vi "IMU RECORDER_AU_2024_v2.vi"() -> ()   [LabVIEW 2021]
uses:
  IMU data typedef.ctl
  <vilib>/Utility/sysdir.llb/System Directory Type.ctl
panel:
  out "TDMS REC!":bool
  in  "Run":bool caption="Run deluje le ob zagonu programa,\nda se zagotovi, da najprej izbereš port.\nÈe program ustaviš s tipko stop, moraš \nza ponoven zagon program še enkrat odpret."
  out "RT REC ID":i32
  in  "Tab Control 2":T1(tab)
  out "LostPackets":cluster{"f":dbl, "f":dbl}(graph)={"f"=1.0, "f"=1.0}
  out "LPR":cluster{dbl, dbl}(graph)={100.0, 100.0}
  out "BATT":cluster{"Ubat 1":dbl, "Ubat 2":dbl}(graph)
  out "Ubat 1":dbl
  out "IMU Temp 1":dbl=25.0
  out "DATA 1":string
  out "Stop IMU 1":bool
  in  "IMU port 1":u16=1235
  in  "T=last value, F=zero 1L":bool=TRUE
  out "Timeout 1":bool=TRUE
  out "IMU1 - 6D":refnum<k16>
  out "IMU DATA 1":T2
  out "IMU DATA 2":T2
  in  "IMU port 2":u16=2000
  out "DATA 2":string
  out "IMU2 - 6D":refnum<k16>
  in  "T=last value, F=zero 1L 2":bool=TRUE caption="T=last value, F=zero 1L"
  out "Timeout 2":bool=TRUE
  out "Stop IMU 2":bool
  out "LiPo MIN":dbl=3.4
  out "LiPo NOM":dbl=3.7
  out "F1":bool
  out "A1":bool=TRUE
  in  "stop 1":bool
  in  "stop 2":bool
  out "IMU Temp 2":dbl=25.0
  out "Ubat 2":dbl
  out "F2":bool
  out "A2":bool=TRUE
  out "GYRO 2":T3(graph)={"AVG(X,N)"=-1.87176, "AVG(X,N)"=2.10976, "AVG(X,N)"=1.55397}
  out "ACC 2":T3(graph)={"AVG(X,N)"=-0.0248636, "AVG(X,N)"=-0.031232, "AVG(X,N)"=0.0110239}
  out "GYRO 1":T3(graph)={"AVG(X,N)"=-1.87176, "AVG(X,N)"=1.48327, "AVG(X,N)"=2.96304}
  in  "IMU CHART":bool=TRUE
  in  "CAL IMU2":bool
  out "BIAS 1":T4={"ACCEL-X"=0.0236778, "ACCEL-Y"=0.0366586, "ACCEL-Z"=-0.00184464, "GYRO - X"=1.87176, "GYRO - Y"=-1.48327, "GYRO - Z"=-2.96304, "TIMESTAMP"=0.0}
  out "BIAS 2":T4={"ACCEL-X"=0.0248636, "ACCEL-Y"=0.031232, "ACCEL-Z"=-0.0110239, "GYRO - X"=1.87176, "GYRO - Y"=-2.10976, "GYRO - Z"=-1.55397, "TIMESTAMP"=0.0}
  out "ACC 1":T3(graph)={"AVG(X,N)"=-0.0236778, "AVG(X,N)"=-0.0366586, "AVG(X,N)"=0.00184464}
  in  "CAL IMU1":bool
  in  "N_BIAS_IMU":i32=100
  out "date/time string":string="2024_02_29"
  out "ShrambaLabview":path=path "C:/Users/marko/TDMS"
  out "Lokacija shranjevanja":path=path "C:/Users/marko/TDMS/2024_02_29"
  in  "sample time":u32=5
  out "LV TimeStamp":i32=16582790
  out "sample ID":i32=109936
  out "ovd":bool
  out "Seconds":i32=550 format="%.2f"
  out "REC FileName":string="IMU-06-06-18-13-48.tdms"
  out "TMP File Name":string="D-02-29-11-54-17.tdms"
  in  "RECORD":bool
  # "FSFV TAPING @ AU 2021 v2"
  # "IP address:  10.10.4.99"
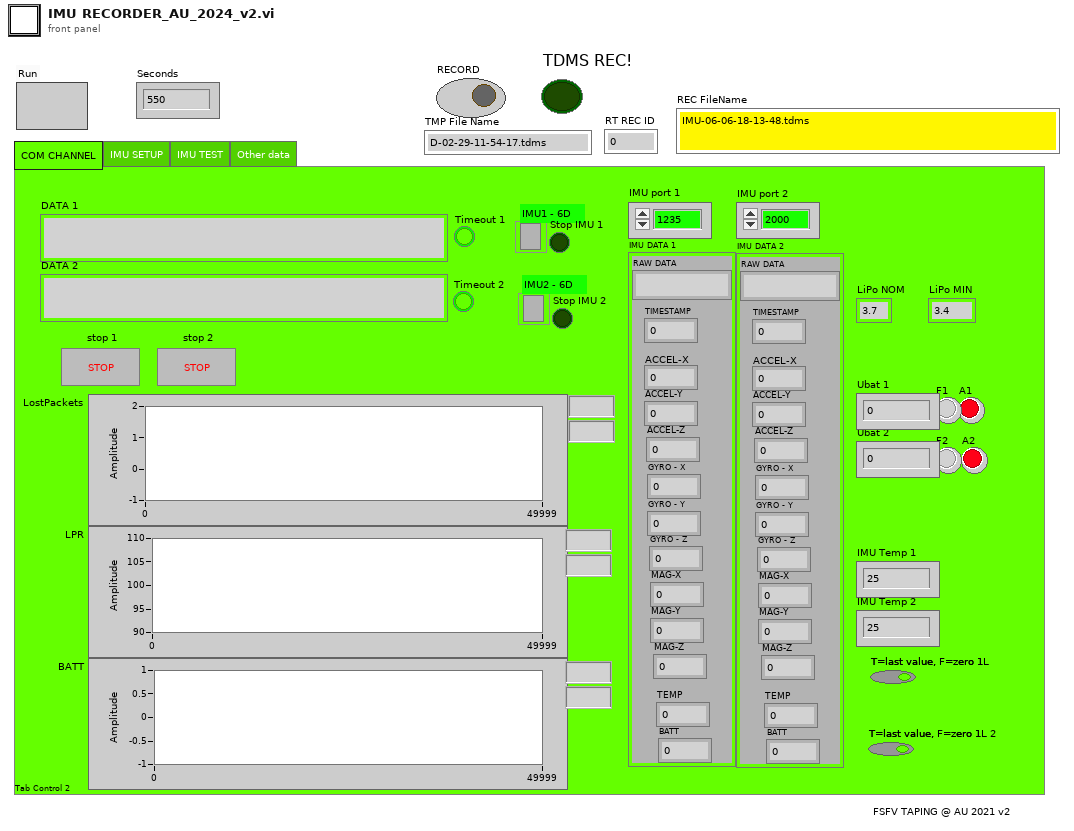
[diagram p1: front panel]
types:
  T1 = enum32{"COM CHANNEL", "IMU SETUP", "IMU TEST", "Other data"}
  T2 = typedef "IMU data typedef.ctl" = cluster{"ACCEL-X":dbl, "ACCEL-Y":dbl, "ACCEL-Z":dbl, "GYRO - X":dbl, "GYRO - Y":dbl, "GYRO - Z":dbl, "MAG-Z":dbl, "MAG-Y":dbl, "MAG-X":dbl, "TEMP":dbl, "BATT":dbl, "RAW DATA":string, "TIMESTAMP":dbl}
  T3 = cluster{"AVG(X,N)":dbl, "AVG(X,N)":dbl, "AVG(X,N)":dbl}
  T4 = cluster{"ACCEL-X":dbl, "ACCEL-Y":dbl, "ACCEL-Z":dbl, "GYRO - X":dbl, "GYRO - Y":dbl, "GYRO - Z":dbl, "TIMESTAMP":dbl}
  T5 = typedef "System Directory Type.ctl" = i32
  T6 = cluster{"ACCEL-X":dbl, "ACCEL-Y":dbl, "ACCEL-Z":dbl}
  T7 = cluster{"GYRO - X":dbl, "GYRO - Y":dbl, "GYRO - Z":dbl}
  T8 = cluster{"AVG(X,N)":dbl, "AVG(X,N)":dbl, dbl, "AVG(X,N)":dbl, "AVG(X,N)":dbl, "AVG(X,N)":dbl, "y":dbl}
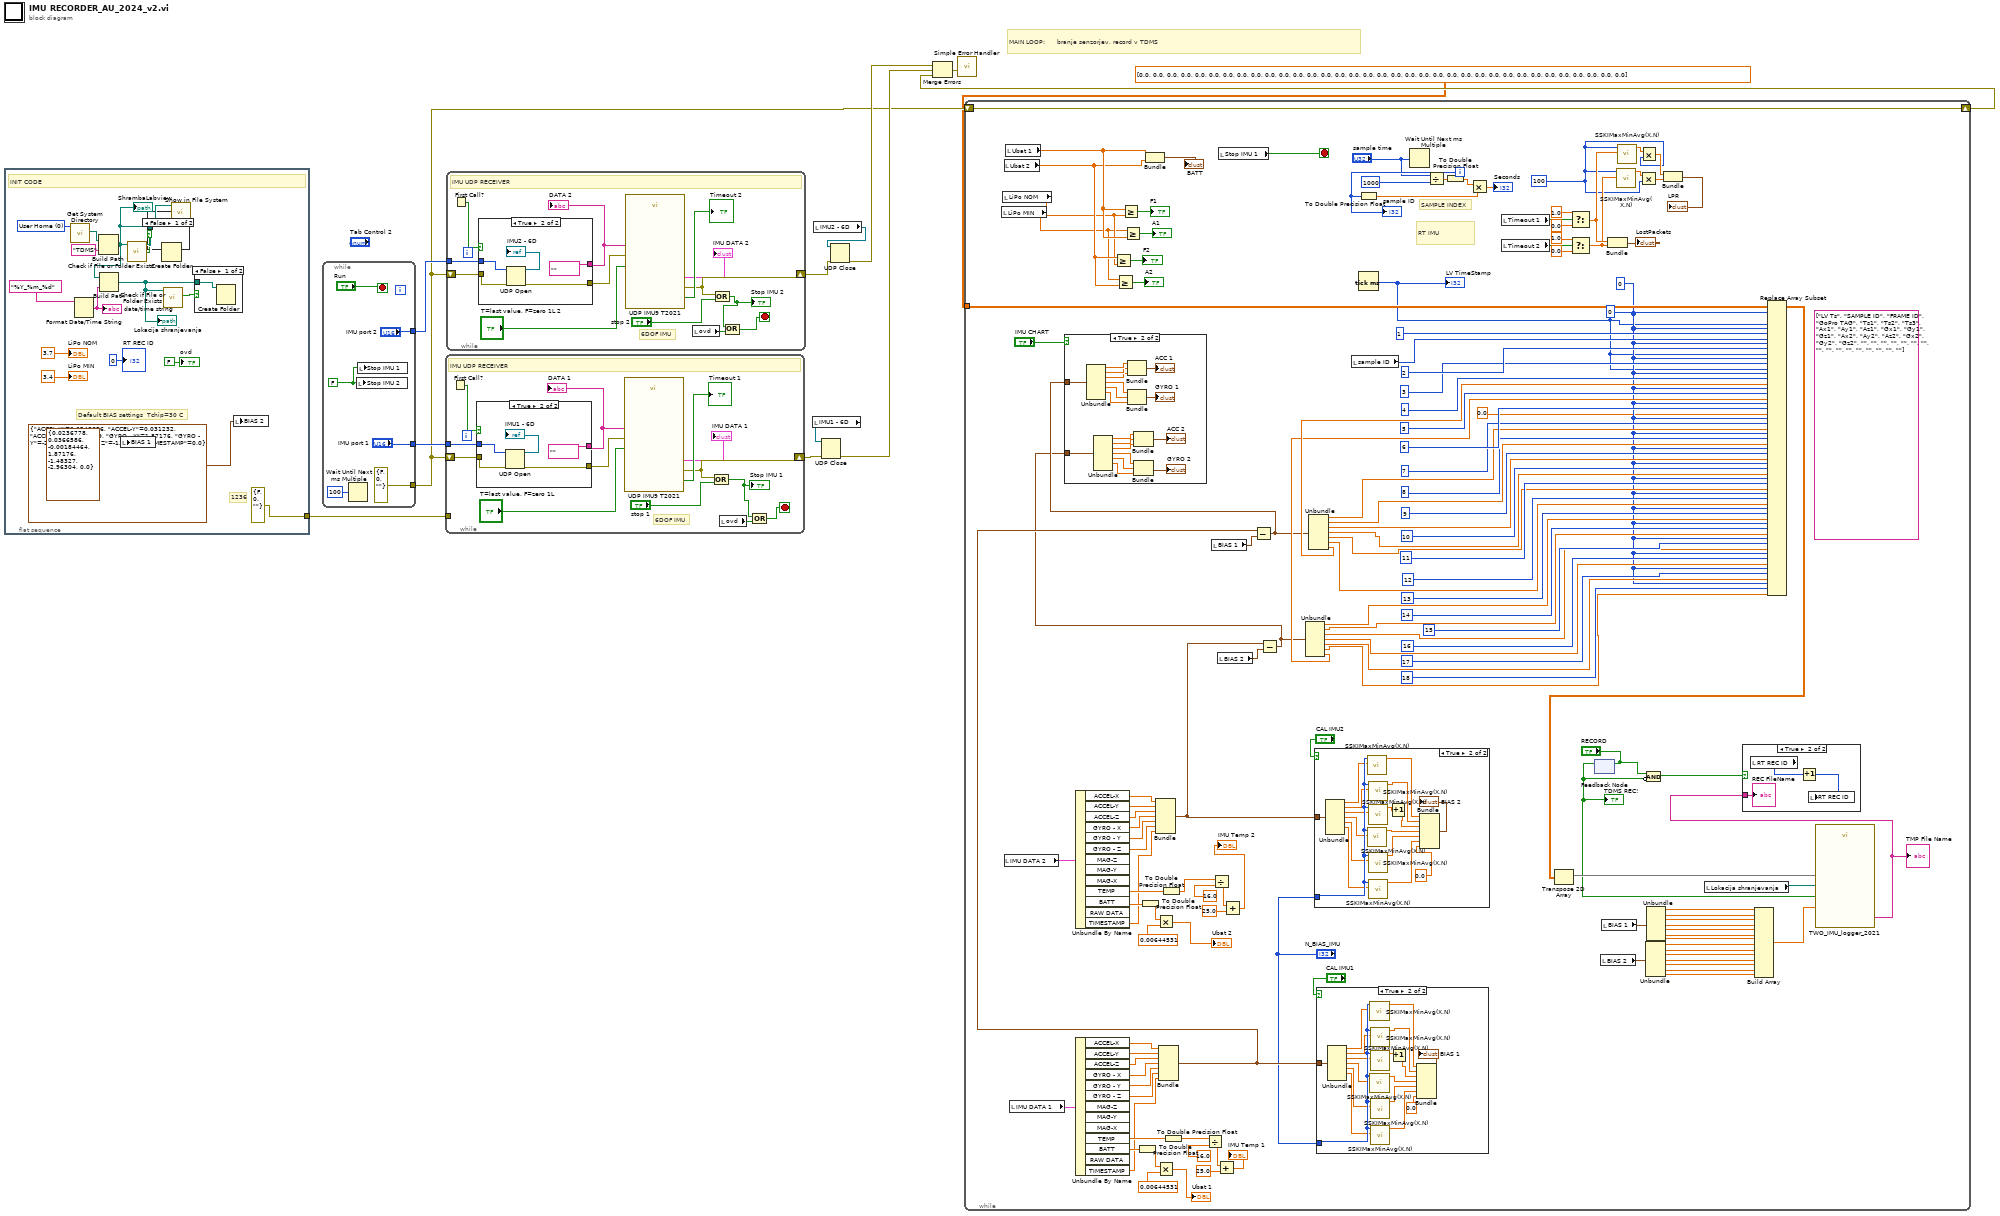
[diagram p0: block diagram]
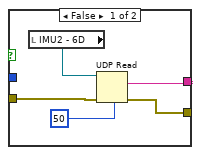
[diagram p2: hidden frame]
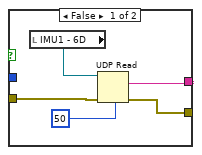
[diagram p9: hidden frame]
diagram:
  # "MAIN LOOP:      branje senzorjev, record v TDMS"
  n1 = flat-sequence {
    tunnel: [errorcluster {"status"=FALSE, "code"=0, "source"=""} ("error constant")] -> w8
    frame #0 {
      w17 = T5 0 items=["User Home"=0, "User Desktop"=1, "User Documents"=2, "User Application Data"=3, "User Preferences"=4, "User Temporary"=5, "Public Documents"=6, "Public Application Data"=7, "Public Preferences"=8, "Public Cache"=13, "System Core Libraries"=9, "System Installed Libraries"=10, "Application Files"=11, "Boot Volume Root"=12] ("system directory type")
      # "1236"
      # "Default BIAS settings  Tchip=30 C"
      # "1235"
      # "INIT CODE"
      n2 = call <vilib>:"Get System Directory.vi"("system directory type"=w17) -> ("system directory"=w19:path)  [unwired: 10 in]
      n3 = Format Date/Time String(time format string (%c)="%Y_%m_%d") -> (date/time string=w21:string)  [unwired: 2 in]
      "date/time string" <- w21
      n4 = Build Path(base path=w19, name or relative path="TDMS") -> (appended path=w24:path)
      "ShrambaLabview" <- w24
      n5 = Build Path(base path=w24, name or relative path=w21) -> (appended path=w23:path)
      "Lokacija shranjevanja" <- w23
      n6 = local write "BIAS 1"(T4 {"ACCEL-X"=0.0236778, "ACCEL-Y"=0.0366586, "ACCEL-Z"=-0.00184464, "GYRO - X"=1.87176, "GYRO - Y"=-1.48327, "GYRO - Z"=-2.96304, "TIMESTAMP"=0.0} ("output cluster")) -> ()
      n7 = call <vilib>:"Check if File or Folder Exists.vi"("path"=w24) -> ("file or folder exists?"=w18:bool, "dup path"=w20:path)  [unwired: 8 in, 1 out]
      n8 = case shown="False" w18 {
        tunnel: w20 -> [_ _]
        frame False {
        }
        frame True {
        }
      }
      n9 = Create Folder() -> ()  [unwired: 3 in, 3 out]
      n10 = call <vilib>:"Check if File or Folder Exists.vi"("path"=w23) -> ("file or folder exists?"=w22:bool)  [unwired: 8 in, 2 out]
      n11 = call <vilib>:"Show in File System.vi"("file or directory path"=w24) -> ()  [unwired: 10 in, 1 out]
      n12 = case shown="False" w22 {
        tunnel: w23 -> [w31 _]
        frame False {
          n13 = Create Folder(path (use dialog)=w31) -> ()  [unwired: 2 in, 3 out]
        }
        frame True {
        }
      }
      n14 = local write "BIAS 2"(T4 {"ACCEL-X"=0.0248636, "ACCEL-Y"=0.031232, "ACCEL-Z"=-0.0110239, "GYRO - X"=1.87176, "GYRO - Y"=-2.10976, "GYRO - Z"=-1.55397, "TIMESTAMP"=0.0} ("output cluster")) -> ()
      "LiPo NOM" <- 3.7 ("LiPo MIN")
      "LiPo MIN" <- 3.4 ("LiPo MIN")
      "RT REC ID" <- 0 ("Trig sample ID")
      "ovd" <- FALSE ("ovd")
    }
  }
  n15 = while {
    tunnel: [errorcluster {"status"=FALSE, "code"=0, "source"=""} ("error constant")] -> w2
    tunnel: ["IMU port 1"] -> w10
    tunnel: ["IMU port 2"] -> w4
    stop <- "Run" stop-if-true
    w32 = FALSE ("Stopping...")
    n16 = Wait Until Next ms Multiple(millisecond multiple=u32 100) -> ()  [unwired: 1 out]
    n17 = local write "Stop IMU 2"(w32) -> ()
    n18 = local write "Stop IMU 1"(w32) -> ()
  }
  n19 = while {
    tunnel: w10 -> [w48]
    shift-right: [w45] -> w11
    shift-left: w2 -> [w47]
    tunnel: w8 -> [_]
    stop <- w39 stop-if-true
    # "6DOF IMU"
    # "IMU UDP RECEIVER"
    n20 = First Call?() -> (First Call?: T/F=w49:bool)
    n21 = case shown="True" w49 {
      tunnel: w48 -> [_ w60]
      tunnel: w47 -> [w53 w58]
      tunnel: [w52 w57] -> w43
      tunnel: [w51 "" ("data out")] -> w44
      frame False {
        n22 = local read "IMU1 - 6D"() -> (w55:refnum<k16>)
        n23 = UDP Read(connection ID=w55, timeout ms (25000)=50, 8:w53) -> (data out=w51:string, error out=w52:errorcluster)  [unwired: 4 out]
      }
      frame True {
        n24 = UDP Open(8:w58, 11:w60) -> (port=→"IMU1 - 6D":refnum<k16>, 0:w57:errorcluster)  [unwired: 3 in, 1 out]
      }
    }
    "DATA 1" <- w44
    n25 = call "UDP IMU9 T2021.vi"("T=last value, F=zero"="T=last value, F=zero 1L", "Error In"=w43, "data in"=w44) -> ("Error Out"=w45:errorcluster, "Data Out"=→"IMU DATA 1":T2, "Timeout"=→"Timeout 1":bool)  [unwired: 6 in]
    n26 = Compound Arithmetic op=OR(w45, "stop 1") -> (w38:bool)
    "Stop IMU 1" <- w38
    n27 = local read "ovd"() -> (w40:bool)
    n28 = Compound Arithmetic op=OR(w38, w40) -> (w39:bool)
  }
  n29 = while {
    tunnel: w4 -> [w71]
    shift-right: [w68] -> w6
    shift-left: w2 -> [w70]
    stop <- w63 stop-if-true
    # "6DOF IMU"
    # "IMU UDP RECEIVER"
    n30 = First Call?() -> (First Call?: T/F=w72:bool)
    n31 = case shown="True" w72 {
      tunnel: w71 -> [_ w83]
      tunnel: w70 -> [w76 w81]
      tunnel: [w75 w80] -> w66
      tunnel: [w74 "" ("data out")] -> w67
      frame False {
        n32 = local read "IMU2 - 6D"() -> (w78:refnum<k16>)
        n33 = UDP Read(connection ID=w78, timeout ms (25000)=50, 8:w76) -> (data out=w74:string, error out=w75:errorcluster)  [unwired: 4 out]
      }
      frame True {
        n34 = UDP Open(8:w81, 11:w83) -> (port=→"IMU2 - 6D":refnum<k16>, 0:w80:errorcluster)  [unwired: 3 in, 1 out]
      }
    }
    "DATA 2" <- w67
    n35 = call "UDP IMU9 T2021.vi"("T=last value, F=zero"="T=last value, F=zero 1L 2", "Error In"=w66, "data in"=w67) -> ("Error Out"=w68:errorcluster, "Data Out"=→"IMU DATA 2":T2, "Timeout"=→"Timeout 2":bool)  [unwired: 6 in]
    n36 = local read "ovd"() -> (w61:bool)
    n37 = Compound Arithmetic op=OR(w68, "stop 2") -> (w62:bool)
    "Stop IMU 2" <- w62
    n38 = Compound Arithmetic op=OR(w62, w61) -> (w63:bool)
  }
  n39 = local read "IMU1 - 6D"() -> (w12:refnum<k16>)
  n40 = local read "IMU2 - 6D"() -> (w3:refnum<k16>)
  n41 = UDP Close(connection ID=w12, 8:w11) -> (error out=w13:errorcluster)  [unwired: 1 out]
  n42 = UDP Close(connection ID=w3, 8:w6) -> (error out=w5:errorcluster)  [unwired: 1 out]
  n43 = while {
    tunnel: dbl[][] [[0.0, 0.0, 0.0, 0.0, 0.0, 0.0, 0.0, 0.0, 0.0, 0.0, 0.0, 0.0, 0.0, 0.0, 0.0, 0.0, 0.0, 0.0, 0.0, 0.0, 0.0, 0.0, 0.0, 0.0, 0.0, 0.0, 0.0, 0.0, 0.0, 0.0, 0.0, 0.0, 0.0, 0.0, 0.0]] ("LOG REC data") -> [w223]
    shift-right: [w206] -> w7
    shift-left: w2 -> [w206]
    i -> [w198]
    stop <- w205 stop-if-true
    (unwired) string[] ["LV Ts", "SAMPLE ID", "FRAME ID", "GoPro TAG", "Ts1", "Ts2", "Ts3", "Ax1", "Ay1", "Az1", "Gx1", "Gy1", "Gz1", "Ax2", "Ay2", "Az2", "Gx2", "Gy2", "Gz2", "", "", "", "", "", "", "", "", "", "", "", "", "", "", "", ""] ("channel name(s) in (Untitled)")
    w103 = 100 ("INT_ N")
    w99 = 0 ("disabled index (row)")
    # "SAMPLE INDEX"
    # "RT IMU"
    n44 = local read "LiPo MIN"() -> (w94:dbl)
    n45 = local read "LiPo NOM"() -> (w95:dbl)
    n46 = local read "Ubat 2"() -> (w96:dbl)
    n47 = local read "IMU DATA 2"() -> (w162:T2)
    n48 = local read "Ubat 1"() -> (w100:dbl)
    n49 = local read "IMU DATA 1"() -> (w175:T2)
    n50 = Unbundle By Name(w162) -> ("ACCEL-X"=w168:dbl, "ACCEL-Y"=w167:dbl, "ACCEL-Z"=w166:dbl, "GYRO - X"=w163:dbl, "GYRO - Y"=w164:dbl, "GYRO - Z"=w165:dbl, "TEMP"=w161:dbl, "BATT"=w160:dbl, "TIMESTAMP"=w152:dbl)  [unwired: 4 out]
    n51 = Unbundle By Name(w175) -> ("ACCEL-X"=w169:dbl, "ACCEL-Y"=w170:dbl, "ACCEL-Z"=w171:dbl, "GYRO - X"=w174:dbl, "GYRO - Y"=w173:dbl, "GYRO - Z"=w172:dbl, "TEMP"=w182:dbl, "BATT"=w183:dbl, "TIMESTAMP"=w153:dbl)  [unwired: 4 out]
    n52 = Greater Or Equal?(x=w96, y=w95) -> (x >= y?=→"F2":bool)
    n53 = Greater Or Equal?(x=w94, y=w96) -> (x >= y?=→"A2":bool)
    n54 = Greater Or Equal?(x=w100, y=w95) -> (x >= y?=→"F1":bool)
    n55 = Greater Or Equal?(x=w94, y=w100) -> (x >= y?=→"A1":bool)
    n56 = To Double Precision Float(number=w183) -> (double precision float=w200:dbl)
    n57 = To Double Precision Float(number=w160) -> (double precision float=w158:dbl)
    n58 = Bundle("Ubat 1"=w100, "Ubat 2"=w96) -> (→"BATT":cluster{"Ubat 1":dbl, "Ubat 2":dbl})  [unwired: 1 in]
    n59 = Bundle("ACCEL-X"=w168, "ACCEL-Y"=w167, "ACCEL-Z"=w166, "GYRO - X"=w163, "GYRO - Y"=w164, "GYRO - Z"=w165, "TIMESTAMP"=w152) -> (w88:T4)  [unwired: 1 in]
    n60 = Multiply(x=w158, y=0.00644531) -> (x*y=→"Ubat 2":dbl)
    n61 = Multiply(x=w200, y=0.00644531) -> (x*y=→"Ubat 1":dbl)
    n62 = Bundle("ACCEL-X"=w169, "ACCEL-Y"=w170, "ACCEL-Z"=w171, "GYRO - X"=w174, "GYRO - Y"=w173, "GYRO - Z"=w172, "TIMESTAMP"=w153) -> (w93:T4)  [unwired: 1 in]
    n63 = To Double Precision Float(number=w161) -> (double precision float=w114:dbl)
    n64 = To Double Precision Float(number=w182) -> (double precision float=w199:dbl)
    n65 = Divide(x=w199, y=16.0) -> (x/y=w203:dbl)
    n66 = local read "BIAS 1"() -> (w132:T4)
    n67 = Divide(x=w114, y=16.0) -> (x/y=w155:dbl)
    n68 = Add(x=w203, y=25.0) -> (x+y=→"IMU Temp 1":dbl)
    n69 = local read "BIAS 2"() -> (w131:T4)
    n70 = local read "Stop IMU 1"() -> (w205:bool)
    n71 = Add(x=w155, y=25.0) -> (x+y=→"IMU Temp 2":dbl)
    n72 = Subtract(x=w93, y=w132) -> (x-y=w85:T4)
    n73 = Subtract(x=w88, y=w131) -> (x-y=w84:T4)
    n74 = case shown="True" "IMU CHART" {
      tunnel: w85 -> [_ w271]
      tunnel: w84 -> [_ w264]
      frame False {
      }
      frame True {
        n75 = Unbundle(w271) -> ("ACCEL-X"=w277:dbl, "ACCEL-Y"=w276:dbl, "ACCEL-Z"=w275:dbl, "GYRO - X"=w274:dbl, "GYRO - Y"=w273:dbl, "GYRO - Z"=w272:dbl)  [unwired: 1 out]
        n76 = Unbundle(w264) -> ("ACCEL-X"=w265:dbl, "ACCEL-Y"=w266:dbl, "ACCEL-Z"=w267:dbl, "GYRO - X"=w268:dbl, "GYRO - Y"=w269:dbl, "GYRO - Z"=w270:dbl)  [unwired: 1 out]
        n77 = Bundle("ACCEL-X"=w277, "ACCEL-Y"=w276, "ACCEL-Z"=w275) -> (→"ACC 1":T6)  [unwired: 1 in]
        n78 = Bundle("GYRO - X"=w274, "GYRO - Y"=w273, "GYRO - Z"=w272) -> (→"GYRO 1":T7)  [unwired: 1 in]
        n79 = Bundle("ACCEL-X"=w265, "ACCEL-Y"=w266, "ACCEL-Z"=w267) -> (→"ACC 2":T6)  [unwired: 1 in]
        n80 = Bundle("GYRO - X"=w268, "GYRO - Y"=w269, "GYRO - Z"=w270) -> (→"GYRO 2":T7)  [unwired: 1 in]
      }
    }
    n81 = Unbundle(w84) -> ("ACCEL-X"=w144:dbl, "ACCEL-Y"=w142:dbl, "ACCEL-Z"=w140:dbl, "GYRO - X"=w138:dbl, "GYRO - Y"=w136:dbl, "GYRO - Z"=w134:dbl, "TIMESTAMP"=w133:dbl)
    n82 = Unbundle(w85) -> ("ACCEL-X"=w151:dbl, "ACCEL-Y"=w150:dbl, "ACCEL-Z"=w149:dbl, "GYRO - X"=w148:dbl, "GYRO - Y"=w147:dbl, "GYRO - Z"=w146:dbl, "TIMESTAMP"=w145:dbl)
    n83 = case shown="True" "CAL IMU2" {
      tunnel: "N_BIAS_IMU" -> [_ w241]
      tunnel: w88 -> [_ w234]
      frame False {
      }
      frame True {
        n84 = Unbundle(w234) -> ("ACCEL-X"=w240:dbl, "ACCEL-Y"=w239:dbl, "ACCEL-Z"=w238:dbl, "GYRO - X"=w237:dbl, "GYRO - Y"=w236:dbl, "GYRO - Z"=w235:dbl)  [unwired: 1 out]
        n85 = call "SSKIMaxMinAvg(X,N).vi"("X"=w240, "INT_ N"=w241) -> ("AVG(X,N)"=w233:dbl)  [unwired: 5 in, 4 out]
        n86 = call "SSKIMaxMinAvg(X,N).vi"("X"=w237, "INT_ N"=w241) -> ("AVG(X,N)"=w231:dbl)  [unwired: 5 in, 4 out]
        n87 = call "SSKIMaxMinAvg(X,N).vi"("X"=w239, "INT_ N"=w241) -> ("AVG(X,N)"=w232:dbl)  [unwired: 5 in, 4 out]
        n88 = call "SSKIMaxMinAvg(X,N).vi"("X"=w238, "INT_ N"=w241) -> ("AVG(X,N)"=w226:dbl)  [unwired: 5 in, 4 out]
        n89 = call "SSKIMaxMinAvg(X,N).vi"("X"=w236, "INT_ N"=w241) -> ("AVG(X,N)"=w230:dbl)  [unwired: 5 in, 4 out]
        n90 = call "SSKIMaxMinAvg(X,N).vi"("X"=w235, "INT_ N"=w241) -> ("AVG(X,N)"=w229:dbl)  [unwired: 5 in, 4 out]
        n91 = Increment(x=w226) -> (x+1=w225:dbl)
        n92 = Bundle("AVG(X,N)"=w233, "AVG(X,N)"=w232, w225, "AVG(X,N)"=w231, "AVG(X,N)"=w230, "AVG(X,N)"=w229, "y"=0.0) -> (→"BIAS 2":T8)  [unwired: 1 in]
      }
    }
    n93 = case shown="True" "CAL IMU1" {
      tunnel: "N_BIAS_IMU" -> [_ w258]
      tunnel: w93 -> [_ w251]
      frame False {
      }
      frame True {
        n94 = Unbundle(w251) -> ("ACCEL-X"=w257:dbl, "ACCEL-Y"=w256:dbl, "ACCEL-Z"=w255:dbl, "GYRO - X"=w254:dbl, "GYRO - Y"=w253:dbl, "GYRO - Z"=w252:dbl)  [unwired: 1 out]
        n95 = call "SSKIMaxMinAvg(X,N).vi"("X"=w257, "INT_ N"=w258) -> ("AVG(X,N)"=w250:dbl)  [unwired: 5 in, 4 out]
        n96 = call "SSKIMaxMinAvg(X,N).vi"("X"=w254, "INT_ N"=w258) -> ("AVG(X,N)"=w248:dbl)  [unwired: 5 in, 4 out]
        n97 = call "SSKIMaxMinAvg(X,N).vi"("X"=w256, "INT_ N"=w258) -> ("AVG(X,N)"=w249:dbl)  [unwired: 5 in, 4 out]
        n98 = call "SSKIMaxMinAvg(X,N).vi"("X"=w255, "INT_ N"=w258) -> ("AVG(X,N)"=w243:dbl)  [unwired: 5 in, 4 out]
        n99 = call "SSKIMaxMinAvg(X,N).vi"("X"=w253, "INT_ N"=w258) -> ("AVG(X,N)"=w247:dbl)  [unwired: 5 in, 4 out]
        n100 = call "SSKIMaxMinAvg(X,N).vi"("X"=w252, "INT_ N"=w258) -> ("AVG(X,N)"=w246:dbl)  [unwired: 5 in, 4 out]
        n101 = Increment(x=w243) -> (x+1=w242:dbl)
        n102 = Bundle("AVG(X,N)"=w250, "AVG(X,N)"=w249, w242, "AVG(X,N)"=w248, "AVG(X,N)"=w247, "AVG(X,N)"=w246, "y"=0.0) -> (→"BIAS 1":T8)  [unwired: 1 in]
      }
    }
    n103 = local read "sample ID"() -> (w181:i32)
    n104 = Tick Count (ms)() -> (millisecond timer value=w91:u32)
    "LV TimeStamp" <- w91
    n105 = To Double Precision Float(number=w198) -> (double precision float=w197:dbl)
    n106 = Wait Until Next ms Multiple(millisecond multiple="sample time") -> ()  [unwired: 1 out]
    n107 = Divide(x="sample time", y=i64 1000) -> (x/y=w196:dbl)
    n108 = To Double Precision Float(number=w196) -> (double precision float=w195:dbl)
    n109 = Multiply(x=w195, y=w197) -> (x*y=→"Seconds":dbl)
    n110 = local read "Timeout 1"() -> (w187:bool)
    n111 = local read "Timeout 2"() -> (w112:bool)
    n112 = Select(t=1.0, s=w187, f=0.0) -> (s? t:f=w108:dbl)
    n113 = Select(t=1.0, s=w112, f=0.0) -> (s? t:f=w107:dbl)
    n114 = feedback-in #1("RECORD") -> ()
    n115 = feedback #1() -> (w177:bool)  [unwired: 1 in]
    "TDMS REC!" <- w177
    n116 = local read "BIAS 2"() -> (w122:T4)
    n117 = local read "BIAS 1"() -> (w130:T4)
    n118 = Bundle("f"=w108, "f"=w107) -> (→"LostPackets":cluster{"f":dbl, "f":dbl})  [unwired: 1 in]
    n119 = call "SSKIMaxMinAvg(X,N).vi"("X"=w107, "INT_ N"=w103) -> ("AVG(X,N)"=w186:dbl)  [unwired: 5 in, 4 out]
    n120 = call "SSKIMaxMinAvg(X,N).vi"("X"=w108, "INT_ N"=w103) -> ("AVG(X,N)"=w106:dbl)  [unwired: 5 in, 4 out]
    n121 = Multiply(x=w186, y=w103) -> (x*y=w105:dbl)
    n122 = Multiply(x=w106, y=w103) -> (x*y=w104:dbl)
    n123 = Unbundle(w122) -> ("ACCEL-X"=w121:dbl, "ACCEL-Y"=w120:dbl, "ACCEL-Z"=w119:dbl, "GYRO - X"=w118:dbl, "GYRO - Y"=w117:dbl, "GYRO - Z"=w116:dbl, "TIMESTAMP"=w115:dbl)
    n124 = Compound Arithmetic op=AND("RECORD", invert w177) -> (w189:bool)
    n125 = Unbundle(w130) -> ("ACCEL-X"=w129:dbl, "ACCEL-Y"=w128:dbl, "ACCEL-Z"=w127:dbl, "GYRO - X"=w126:dbl, "GYRO - Y"=w125:dbl, "GYRO - Z"=w124:dbl, "TIMESTAMP"=w123:dbl)
    n126 = Bundle(w104, w105) -> (→"LPR":cluster{dbl, dbl})  [unwired: 1 in]
    n127 = local read "Lokacija shranjevanja"() -> (w178:path)
    n128 = Build Array(w129, w128, w127, w126, w125, w124, w123, w121, w120, w119, w118, w117, w116, w115) -> (w176:dbl[])
    n129 = Replace Array Subset(array=w223, new element #1=w91, index (row) #1=w99, index (col) #1=0 ("index"), new element #2=w181, index (row) #2=w99, index (col) #2=1 ("index"), new element #3=w91, index (row) #3=w99, index (col) #3=2 ("index"), new element #4=w91, index (row) #4=w99, index (col) #4=3 ("index"), new element #5=w145, index (row) #5=w99, index (col) #5=4 ("index"), new element #6=w133, index (row) #6=w99, index (col) #6=5 ("index"), new element #7=0.0 ("new element/subarray"), index (row) #7=w99, index (col) #7=6 ("index"), new element #8=w151, index (row) #8=w99, index (col) #8=7 ("index"), new element #9=w150, index (row) #9=w99, index (col) #9=8 ("index"), new element #10=w149, index (row) #10=w99, index (col) #10=9 ("index"), new element #11=w148, index (row) #11=w99, index (col) #11=10 ("index"), new element #12=w147, index (row) #12=w99, index (col) #12=11 ("index"), new element #13=w146, index (row) #13=w99, index (col) #13=12 ("index"), new element #14=w144, index (row) #14=w99, index (col) #14=13 ("index"), new element #15=w142, index (row) #15=w99, index (col) #15=14 ("index"), new element #16=w140, index (row) #16=w99, index (col) #16=15 ("index"), new element #17=w138, index (row) #17=w99, index (col) #17=16 ("index"), new element #18=w136, index (row) #18=w99, index (col) #18=17 ("index"), new element #19=w134, index (row) #19=w99, index (col) #19=18 ("index")) -> (w221:dbl[][])
    n130 = Transpose 2D Array(2D array=w221) -> (transposed array=w220:dbl[][])
    n131 = call "TWO_IMU_logger_2021.vi"("PARAMETERS"=w176, "Folder"=w178, "LOG"=w177, "DATA"=w220) -> ("FileName"=w188:string)  [unwired: 7 in]
    "TMP File Name" <- w188
    n132 = case shown="True" w189 {
      tunnel: w188 -> [_ w261]
      frame False {
      }
      frame True {
        n133 = local read "RT REC ID"() -> (w260:i32)
        n134 = Increment(x=w260) -> (x+1=w259:i32)
        n135 = local write "RT REC ID"(w259) -> ()
        "REC FileName" <- w261
      }
    }
    "sample ID" <- w198
  }
  n136 = Merge Errors(w5, w13, w7) -> (w9:errorcluster)
  n137 = call <vilib>:"Simple Error Handler.vi"("error in (no error)"=w9) -> ()  [unwired: 1 in, 8 out]
